vi "WriteDM_V2.vi"(0 "reference in":refnum<k7>, 1 "nDevId":i32, 2 "MultiDM  Mapping":i32[](array[numeric]), 3 "Voltage Array in":dbl[](array[numeric]), 4 "error in":errorcluster) -> (5 "reference out":refnum<k7>, 7 "error out":errorcluster)   [LabVIEW 2016]
panel:
  out "Pixel Map (-1 to 1)":u16[][](graph)
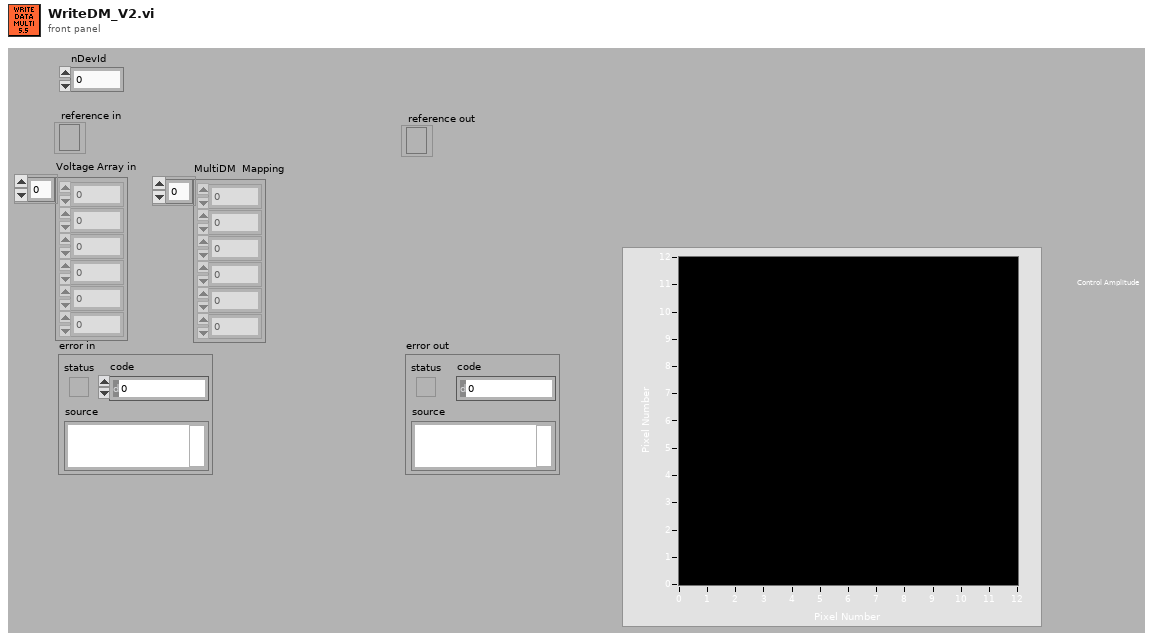
[diagram p1: front panel]
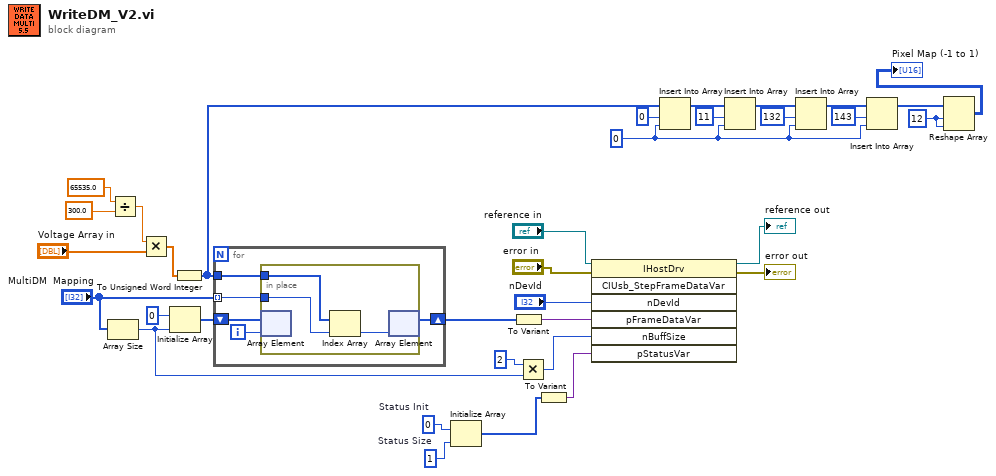
[diagram p0: block diagram]
diagram:
  w2 = u16 0 ("new element/subarray")
  w13 = 12 ("dimension size")
  w22 = 1  # Status Size
  w21 = 0  # Status Init
  n1 = Array Size(array="MultiDM  Mapping") -> (size(s)=w17:i32)
  n2 = Divide(x=65535.0 ("y"), y=300.0 ("x")) -> (x/y=w18:dbl)
  n3 = Multiply(x=w18, y="Voltage Array in") -> (x*y=w29:dbl[])
  n4 = Initialize Array(u16 0 ("element"), w17) -> (w27:u16[])
  n5 = To Unsigned Word Integer(number=w29) -> (unsigned 16bit integer=w1:u16[])
  n6 = for {
    shift-right: [w37] -> w3
    shift-left: w27 -> [w39]
    tunnel: "MultiDM  Mapping" -> [w35] mode=indexing
    tunnel: w1 -> [w38]
    i -> [w36]
    n7 = in-place {
      in-place-border: w38 -> [w41]
      in-place-border: w35 -> [w42]
      n8 = in-place-array #1(w39, w36) -> ()  [unwired: 1 out]
      n9 = Index Array(array=w41, index=w42) -> (element=w40:u16)
      n10 = in-place-array #1(w40) -> (w37:u16[])  [unwired: 1 out]
    }
  }
  n11 = Initialize Array "Initialize Array"(w21, w22) -> (w20:i32[])
  n12 = To Variant(anything=w3) -> (Variant=w32:variant)
  n13 = Multiply(x=2, y=w17) -> (x*y=w15:i32)
  n14 = To Variant(anything=w20) -> (Variant=w19:variant)
  n15 = invoke class="IHostDrv" method="CIUsb_StepFrameDataVar"(reference="reference in", error in="error in", "nDevId"="nDevId", "pFrameDataVar"=w32, "nBuffSize"=w15, "pStatusVar"=w19) -> (reference out=→"reference out":refnum<k7>, error out=→"error out":errorcluster)  [unwired: 1 in, 5 out]
  n16 = Insert Into Array(array=w1, index=0, new element=w2) -> (w7:u16[])
  n17 = Insert Into Array(array=w7, index=11, new element=w2) -> (w9:u16[])
  n18 = Insert Into Array(array=w9, index=132, new element=w2) -> (w11:u16[])
  n19 = Insert Into Array(array=w11, index=143, new element=w2) -> (w4:u16[])
  n20 = Reshape Array(w4, w13, w13) -> (→"Pixel Map (-1 to 1)":u16[][])
